vi "4_4ClusterExercise_BTS.vi"() -> ()   [LabVIEW 2014]
panel:
  out "Small Cluster":cluster{"Boolean":bool, "Slide Value":dbl}
  out "Modified cluster":T1 {"Slide" scale=0.0..10.0}
  in  "Cluster":T1 {"Slide" scale=0.0..10.0}
  out "Boolean":bool
  out "Numeric":dbl
  in  "stop":bool
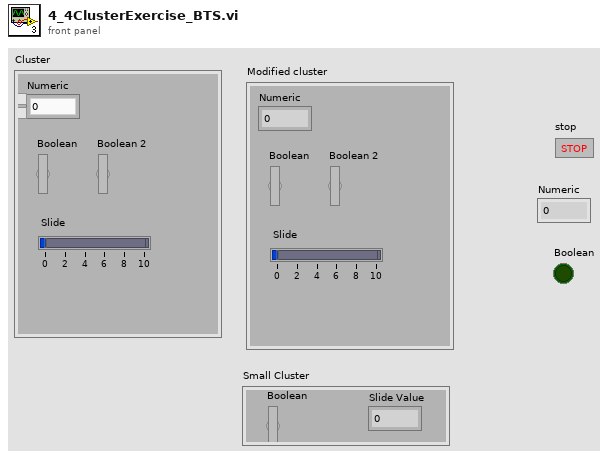
[diagram p1: front panel]
types:
  T1 = cluster{"Numeric":dbl, "Boolean":bool, "Boolean 2":bool, "Slide":dbl}
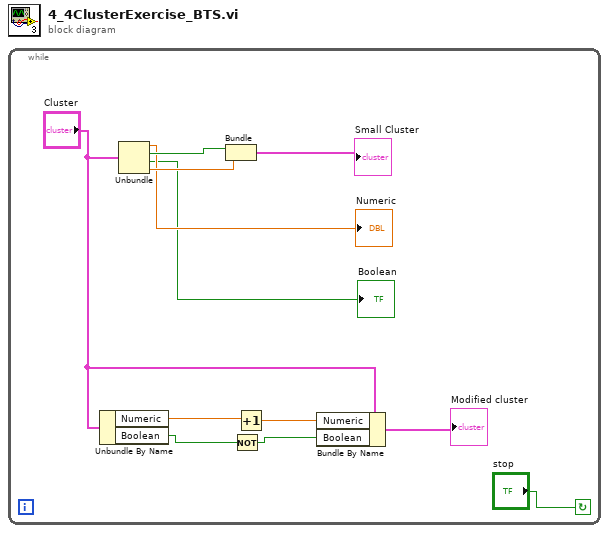
[diagram p0: block diagram]
diagram:
  n1 = while {
    stop <- "stop" continue-if-true
    n2 = Unbundle By Name("Cluster") -> ("Numeric"=w7:dbl, "Boolean"=w4:bool)
    n3 = Unbundle("Cluster") -> ("Numeric"=→"Numeric":dbl, "Boolean"=w11:bool, "Boolean 2"=→"Boolean":bool, "Slide"=w10:dbl)
    n4 = Bundle("Boolean"=w11, "Slide"=w10) -> (→"Small Cluster":cluster{"Boolean":bool, "Slide":dbl})  [unwired: 1 in]
    n5 = Not(x=w4) -> (.not. x?=w3:bool)
    n6 = Increment(x=w7) -> (x+1=w6:dbl)
    n7 = Bundle By Name(cluster="Cluster", "Numeric"=w6, "Boolean"=w3) -> (→"Modified cluster":T1)
  }
